vi "ConnectionClosed.vi"(6 "FinaErrorCode":i32, 8 "error in (no error)":errorcluster, 9 "ClientIP":string, 10 "ConnectionNumber":i32, 11 "TCP_Connections_Controller in":refnum<class "TCP_Connections_Controller.lvclass">) -> (0 "error out":errorcluster, 3 "TCP_Connections_Controller out":refnum<class "TCP_Connections_Controller.lvclass">)   [LabVIEW 2023, in "TCP_Server_Connection_Handler.lvlib" / "TCP_Connections_Controller.lvclass"]
uses:
  TCP_Connections_Controller.lvclass
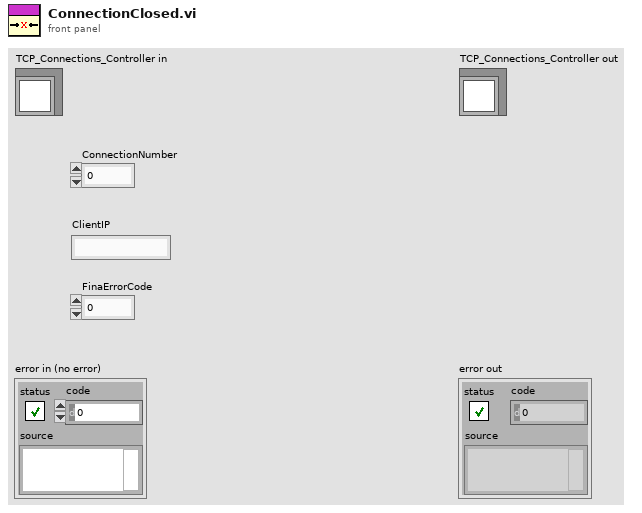
[diagram p1: front panel]
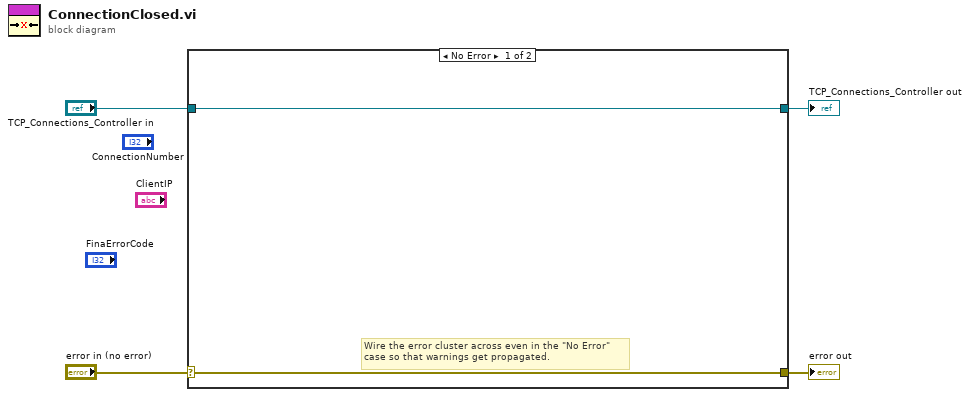
[diagram p0: block diagram]
diagram:
  n1 = case shown="No Error" "error in (no error)" {
    selector: "error in (no error)" -> [w5 w8]
    tunnel: [w5 w8] -> w3
    tunnel: [w6 w7] -> w1
    tunnel: "TCP_Connections_Controller in" -> [w6 w7]
    frame No Error {
      # "Wire the error cluster across even in the \"No Error\"\ncase so that warnings get propagated."
    }
    frame Error {
    }
  }
  "error out" <- w3
  "TCP_Connections_Controller out" <- w1
